vi "Loaded Data Desired to Unique IDs.vi"(9 "Stats":string[][](array[string]), 11 "Data":string[][](array[string])) -> (1 "Stat Out":string[][](array[string]), 3 "Data Out":string[][](array[string]))   [LabVIEW 2013]
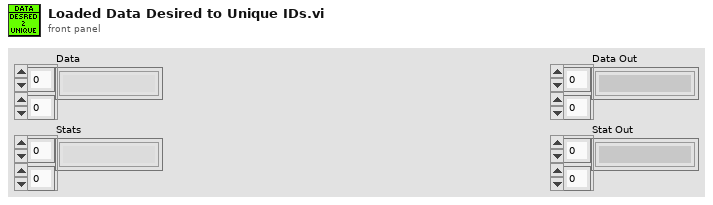
[diagram p1: front panel]
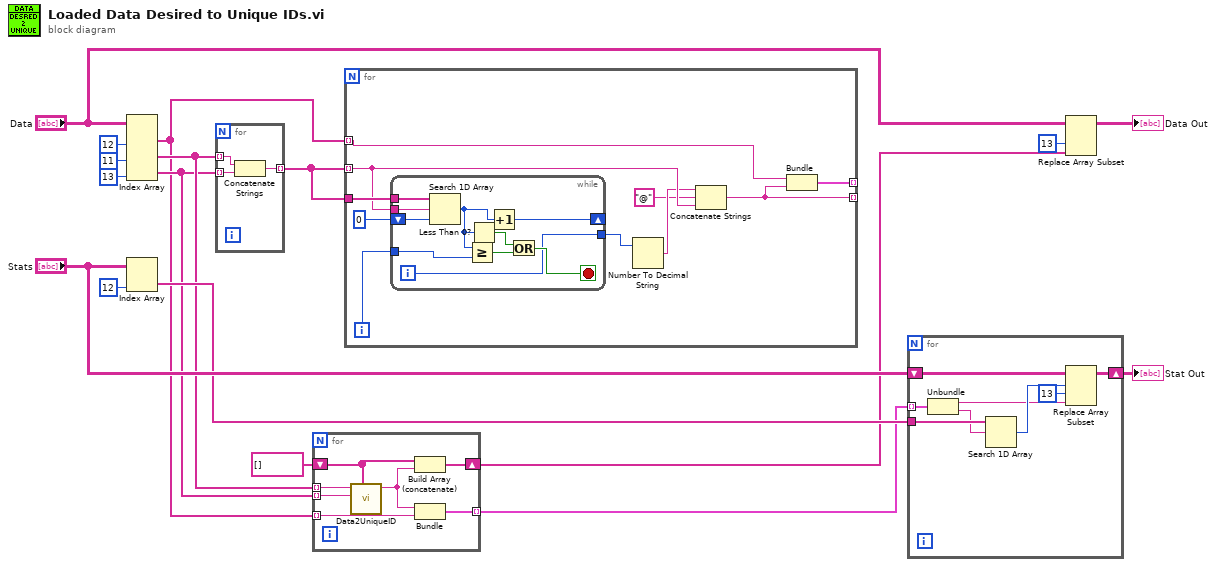
[diagram p0: block diagram]
diagram:
  n1 = Index Array(array="Data", index (col) #1=12 ("disabled index (col)"), index (col) #2=11 ("index (col)"), index (col) #3=13 ("index (col)")) -> (element #1=w1:string[], element #2=w7:string[], element #3=w6:string[])  [unwired: 3 in]
  n2 = Index Array(array="Stats", index (col)=12 ("disabled index (col)")) -> (element=w9:string[])  [unwired: 1 in]
  n3 = for {
    tunnel: w7 -> [w20] mode=indexing
    tunnel: w6 -> [w19] mode=indexing
    tunnel: [w18] -> w14 mode=indexing
    n4 = Concatenate Strings(w20, w19) -> (w18:string)
  }
  n5 = for {
    tunnel: w7 -> [w27] mode=indexing
    tunnel: w6 -> [w26] mode=indexing
    shift-right: [w25] -> w3
    shift-left: string[] [] -> [w24]
    tunnel: w1 -> [w21] mode=indexing
    tunnel: [w23] -> w4 mode=indexing
    n6 = call "Data2UniqueID.vi"("[UniqueID]s"=w24, "ParameterSet"=w26, "Step"=w27) -> ("UniqueID"=w22:string)  [unwired: 8 in]
    n7 = Build Array (concatenate)(w24, w22) -> (w25:string[])
    n8 = Bundle("UniqueID"=w22, w21) -> (w23:cluster{"UniqueID":string, string})  [unwired: 1 in]
  }
  n9 = for {
    tunnel: w1 -> [w30] mode=indexing
    tunnel: w14 -> [w33] mode=indexing
    tunnel: w14 -> [w37]
    tunnel: [w29] -> _ mode=indexing
    tunnel: [w28] -> _ mode=indexing
    i -> [w35]
    n10 = while {
      tunnel: w37 -> [w47]
      tunnel: w33 -> [w46]
      shift-right: [w44] -> _
      shift-left: 0 ("index of element") -> [w45]
      tunnel: w35 -> [w43]
      tunnel: [w38] -> w34
      i -> [w38]
      stop <- w39 stop-if-true
      n11 = Search 1D Array(1D array=w47, element=w46, start index (0)=w45) -> (index of element=w42:i32)
      n12 = Greater Or Equal?(x=w42, y=w43) -> (x >= y?=w40:bool)
      n13 = Less Than 0?(x=w42) -> (x < 0?=w41:bool)
      n14 = Increment(x=w42) -> (x+1=w44:i32)
      n15 = Or(x=w41, y=w40) -> (x .or. y?=w39:bool)
    }
    n16 = Number To Decimal String(number=w34) -> (decimal integer string=w32:string)  [unwired: 1 in]
    n17 = Concatenate Strings(w32, "@" ("string"), w33) -> (w28:string)
    n18 = Bundle(w30, w28) -> (w29:cluster{string, string})  [unwired: 1 in]
  }
  n19 = for {
    tunnel: w4 -> [w55] mode=indexing
    tunnel: w9 -> [w54]
    shift-right: [w52] -> w8
    shift-left: "Stats" -> [w53]
    n20 = Unbundle(w55) -> ("UniqueID"=w49:string, w48:string)
    n21 = Search 1D Array(1D array=w54, element=w48) -> (index of element=w50:i32)  [unwired: 1 in]
    n22 = Replace Array Subset(array=w53, new element=w49, index (row)=w50, index (col)=13 ("disabled index (col)")) -> (w52:string[][])
  }
  "Stat Out" <- w8
  n23 = Replace Array Subset(array="Data", new element=w3, index (col)=13 ("disabled index (col)")) -> (→"Data Out":string[][])  [unwired: 1 in]
